vi "ptspecial.vi"(11 "i ref in":refnum<vi>) -> (3 "i ref out":refnum<vi>)   [LabVIEW 2014, in "Panels.lvlib"]
uses:
  Panels.lvlib
  CSlibraries-extern/DimLVEvent/DimIndicators/DimIndicators.numericArrayType.ctl
  CSlibraries-extern/DimLVEvent/DimIndicators/DimIndicators.lvlib
panel:
  in  "HypCorrTubeBTrap_SetData":T1={"data"=[0.0, 0.0, 0.0, 0.0], "no link"=FALSE, "quality"=1, "timeStamp"=3268846604.91}
  in  "HypCorrTubeATrap_SetData":T1={"data"=[0.0, 0.0, 0.0, 0.0], "no link"=FALSE, "quality"=1, "timeStamp"=3268846604.66}
  in  "HypCorrRingB_SetData":T1={"data"=[0.0, 0.0, 0.0, 0.0], "no link"=FALSE, "quality"=1, "timeStamp"=3268846604.676}
  in  "HypCorrRingA_SetData":T1={"data"=[0.0, 0.0, 0.0, 0.0], "no link"=FALSE, "quality"=1, "timeStamp"=3268846604.644}
  # "********************************************************\nHypCorrRingA = CorrRingPara * (HypEndcapA - HypRing) + HypRing\nHypCorrRingB = CorrRingPara * (HypEndcapB - HypRing) + HypRing\nHypCorrTubeA = CorrTubePara * (HypEndcapA - HypRing) + HypRing\nHypCorrTubeB = CorrTubePara * (HypEndcapB - HypRing) + HypRing\n********************************************************"
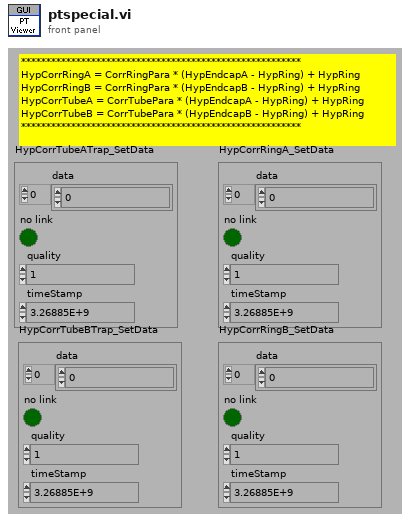
[diagram p1: front panel]
types:
  T1 = typedef "DimIndicators.lvlib/DimIndicators.numericArrayType.ctl" = cluster{"data":dbl[], "no link":bool, "quality":i32, "timeStamp":dbl}
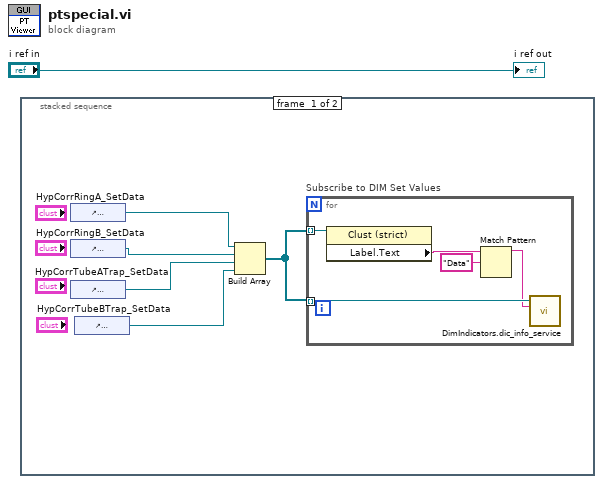
[diagram p0: block diagram]
diagram:
  n1 = stacked-sequence {
    frame #0 {
      n2 = control-ref of="HypCorrRingA_SetData"() -> (w6:refnum<vi>)
      n3 = control-ref of="HypCorrRingB_SetData"() -> (w5:refnum<vi>)
      n4 = control-ref of="HypCorrTubeATrap_SetData"() -> (w4:refnum<vi>)
      n5 = control-ref of="HypCorrTubeBTrap_SetData"() -> (w3:refnum<vi>)
      n6 = Build Array(w6, w5, w4, w3) -> (w2:refnum<vi>[])
      n7 = for "Subscribe to DIM Set Values" {
        tunnel: w2 -> [w7] mode=indexing
        tunnel: w2 -> [w11] mode=indexing
        n8 = property class="Clust (strict)"(reference=w7) -> ("Label.Text"=w10:string)  [unwired: 1 in, 2 out]
        n9 = Match Pattern(string=w10, regular expression="Data") -> (before substring=w8:string)  [unwired: 1 in, 3 out]
        n10 = call "DimIndicators.dic_info_service.vi"("controlRef"=w11, "serviceName"=w8) -> ()  [unwired: 16 in, 2 out]
      }
    }
    frame #1 {
    }
  }
  "i ref out" <- "i ref in"
